vi "SIM BDF Eval Error Core.vi"(0 "outputs":dbl[](array[numeric]), 1 "min float":dbl, 2 "Delta Method Order":i32, 3 "max step ratio":dbl, 5 "step size":dbl, 7 "proposed step size":dbl, 9 "min step size":dbl, 11 "BDF data":T1, 12 "max step size":dbl, 13 "relative tolerance":dbl, 14 "absolute tolerance":dbl) -> (4 "outputs out":dbl[](array[numeric]), 6 "step accepted? out":bool, 8 "proposed step size out":dbl, 10 "proposed max step ratio":dbl, 15 "BDF data out":T1)   [LabVIEW 2017]
uses:
  SIM BDF data.ctl
  SIM Factored Matrix.ctl
  SIM BDF stages.ctl
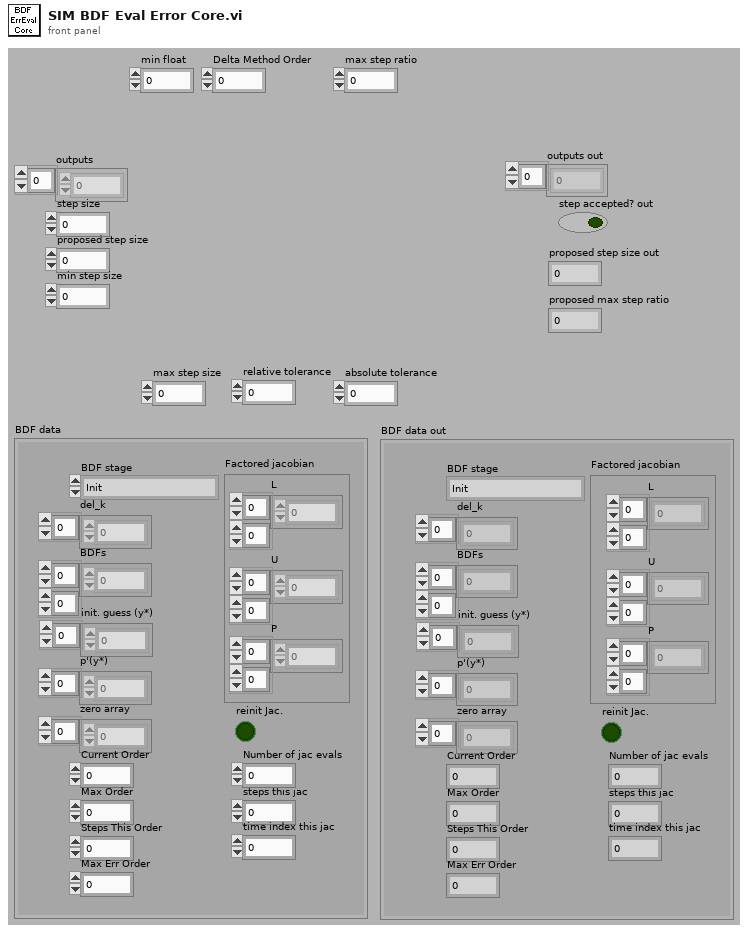
[diagram p1: front panel]
types:
  T1 = typedef "SIM BDF data.ctl" = cluster{"BDFs":dbl[][], "init. guess (y*)":dbl[], "p'(y*)":dbl[], "Factored jacobian":T2, "zero array":dbl[], "reinit Jac.":bool, "BDF stage":T3, "steps this jac":i32, "time index this jac":i32, "Number of jac evals":i32, "del_k":dbl[], "Current Order":i32, "Max Order":i32, "Steps This Order":i32, "Max Err Order":i32}
  T2 = typedef "SIM Factored Matrix.ctl" = cluster{"L":dbl[][], "U":dbl[][], "P":i32[][]}
  T3 = typedef "SIM BDF stages.ctl" = enum16{"Init", "Initial Guess", "Compute Jacobian", "Newton Iteration", "Eval Error", "Choose StepSize", "Reset BDFs"}
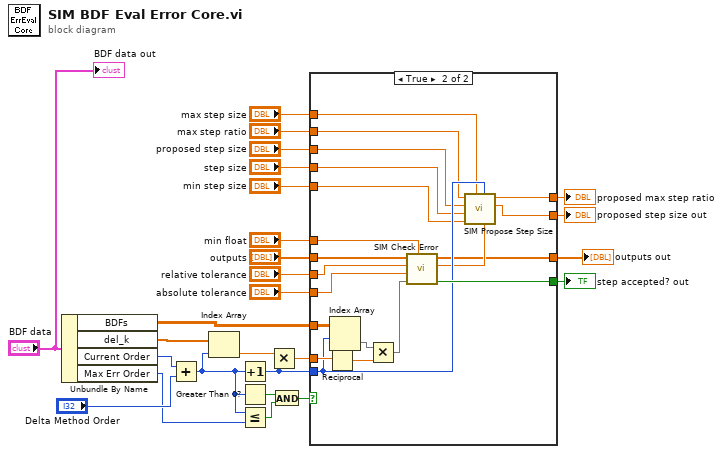
[diagram p0: block diagram]
diagram:
  n1 = Unbundle By Name("BDF data") -> ("BDFs"=w20:dbl[][], "del_k"=w14:dbl[], "Current Order"=w17:i32, "Max Err Order"=w16:i32)
  n2 = Add(x=w17, y="Delta Method Order") -> (x+y=w15:i32)
  n3 = Index Array(array=w14, index=w15) -> (element=w12:dbl)
  n4 = Increment(x=w15) -> (x+1=w13:i32)
  n5 = Greater Than 0?(x=w15) -> (x > 0?=w23:bool)
  n6 = Less Or Equal?(x=w15, y=w16) -> (x <= y?=w19:bool)
  n7 = Multiply(x=w12, y=w13) -> (x*y=w11:dbl)
  n8 = And(x=w23, y=w19) -> (x .and. y?=w22:bool)
  n9 = case shown="True" w22 {
    tunnel: "outputs" -> [w27 w30]
    tunnel: w20 -> [_ w47]
    tunnel: w13 -> [_ w38]
    tunnel: [_ w39] -> w26
    tunnel: [_ w36] -> w25
    tunnel: [_ w37] -> w24
    tunnel: w11 -> [_ w46]
    tunnel: "relative tolerance" -> [_ w42]
    tunnel: "min float" -> [_ w43]
    tunnel: "absolute tolerance" -> [_ w41]
    tunnel: "max step size" -> [_ w35]
    tunnel: "max step ratio" -> [_ w34]
    tunnel: "proposed step size" -> [_ w33]
    tunnel: "step size" -> [_ w32]
    tunnel: "min step size" -> [_ w31]
    tunnel: [w27 w28] -> w1
    frame False {
    }
    frame True {
      n10 = Reciprocal(x=w46) -> (1/x=w45:dbl)
      n11 = Index Array(array=w47, index (row)=w38) -> (element=w44:dbl[])  [unwired: 1 in]
      n12 = Multiply(x=w44, y=w45) -> (x*y=w40:dbl[])
      n13 = call "SIM Check Error.vi"("min float"=w43, "estimated error"=w40, "absolute tolerance"=w41, "relative tolerance"=w42, "Solution"=w30) -> ("within acceptable err?"=w39:bool, "acceptable err/estimated err"=w29:dbl, "Solution Out"=w28:dbl[])  [unwired: 4 out]
      n14 = call "SIM Propose Step Size.vi"("acceptable err/estimated err"=w29, "error order"=w38, "max step size"=w35, "min step size"=w31, "step size"=w32, "proposed step size"=w33, "max step ratio"=w34) -> ("proposed step size out"=w36:dbl, "proposed max step ratio"=w37:dbl)  [unwired: 3 out]
    }
  }
  "step accepted? out" <- w26
  "proposed step size out" <- w25
  "proposed max step ratio" <- w24
  "outputs out" <- w1
  "BDF data out" <- "BDF data"
